vi "EncoderPID.vi"() -> (2 "PID 2 Output":dbl, 3 "PID 1 Output":dbl)   [LabVIEW 2013]
uses:
  <vilib>/addons/control/pid/pid.llb/PID (DBL).vi
  <vilib>/addons/control/pid/NI_PID_pid.lvlib
panel:
  in  "PID gains Shooter Wheels":T1={"proportional gain (Kc)"=1.0, "integral time (Ti, min)"=0.01, "derivative time (Td, min)"=0.0} {"derivative time (Td, min)" format="%.3f"; "integral time (Ti, min)" format="%.3f"; "proportional gain (Kc)" format="%.3f"}
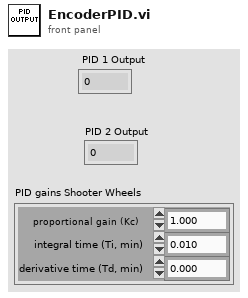
[diagram p1: front panel]
types:
  T1 = cluster{"proportional gain (Kc)":dbl, "integral time (Ti, min)":dbl, "derivative time (Td, min)":dbl}
  T2 = typedef "WPI_EncoderDevRef.ctl" = cluster{"DevStatus":errorcluster, "EncoderIndex":T3, "CounterIndex":T4, "DistancePerCount":dbl, "Decoding Type":T5}
  T3 = typedef "FPGA_EncoderIdx.ctl" = enum8{"Enc 0", "Enc 1", "Enc 2", "Enc 3", "Invalid"}
  T4 = typedef "FPGA_CounterCtrSystemIndex.ctl" = enum8{"Ctr 0", "Ctr 1", "Ctr 2", "Ctr 3", "Ctr 4", "Ctr 5", "Ctr 6", "Ctr 7", "Invalid"}
  T5 = typedef "WPI_EncoderType.ctl" = enum16{"1x", "2x", "4x"}
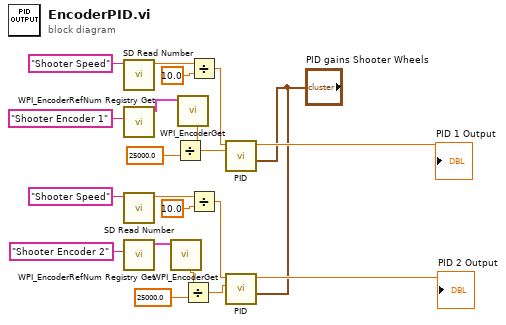
[diagram p0: block diagram]
diagram:
  n1 = call <vilib>:"SD Read Number.vi"("Name"="Shooter Speed") -> ("Numeric"=w16:dbl)  [unwired: 8 in, 2 out]
  n2 = call <vilib>:"WPI_EncoderRefNum Registry Get.vi"("refnum name"="Shooter Encoder 1") -> ("EncoderDevRef"=w18:T2)  [unwired: 9 in, 1 out]
  n3 = call <vilib>:"SD Read Number.vi"("Name"="Shooter Speed") -> ("Numeric"=w12:dbl)  [unwired: 8 in, 2 out]
  n4 = call <vilib>:"WPI_EncoderRefNum Registry Get.vi"("refnum name"="Shooter Encoder 2") -> ("EncoderDevRef"=w20:T2)  [unwired: 9 in, 1 out]
  n5 = call <vilib>:"WPI_EncoderGet.vi"("EncoderDevRef"=w20) -> ("Rate"=w3:dbl)  [unwired: 5 in, 5 out]
  n6 = call <vilib>:"WPI_EncoderGet.vi"("EncoderDevRef"=w18) -> ("Rate"=w7:dbl)  [unwired: 5 in, 5 out]
  n7 = Divide(x=w7, y=25000.0) -> (x/y=w6:dbl)
  n8 = Divide(x=w3, y=25000.0) -> (x/y=w4:dbl)
  n9 = Divide(x=w16, y=10.0) -> (x/y=w14:dbl)
  n10 = Divide(x=w12, y=10.0) -> (x/y=w10:dbl)
  n11 = call-poly <vilib>:"PID.vi"("PID gains"="PID gains Shooter Wheels", "process variable"=w6, "setpoint"=w14) -> ("output"=→"PID 1 Output":dbl)  [unwired: 7 in, 1 out]
  n12 = call-poly <vilib>:"PID.vi"("PID gains"="PID gains Shooter Wheels", "process variable"=w4, "setpoint"=w10) -> ("output"=→"PID 2 Output":dbl)  [unwired: 7 in, 1 out]
